vi "ROI entry-Previous ROI compat-Motor Z check.vi"(8 "error in (no error)":errorcluster, 9 "Proceed":bool=TRUE, 10 "ROI fit info cluster in":T1 {"ROI fit info"."Frame size"."Old" items=["100X100"=100, "128X128"=128, "200X200"=200, "256X256"=256, "512X512"=512, "1024x1024"=1024, "2048x2048"=2048]; "ROI fit info"."Frame size"."New" items=["100X100"=100, "128X128"=128, "200X200"=200, "256X256"=256, "512X512"=512, "1024x1024"=1024, "2048x2048"=2048]}, 11 "Old ROI file path":path) -> (0 "error out":errorcluster, 1 "Proceed":bool, 2 "ROI fit info cluster":T1 {"ROI fit info"."Frame size"."Old" items=["100X100"=100, "128X128"=128, "200X200"=200, "256X256"=256, "512X512"=512, "1024x1024"=1024, "2048x2048"=2048]; "ROI fit info"."Frame size"."New" items=["100X100"=100, "128X128"=128, "200X200"=200, "256X256"=256, "512X512"=512, "1024x1024"=1024, "2048x2048"=2048]}, 3 "Old ROI file path (dup)":path)   [LabVIEW 2017]
uses:
  Typedefs/ROI fitting info cluster.ctl
  Typedefs/Frame Size.ctl
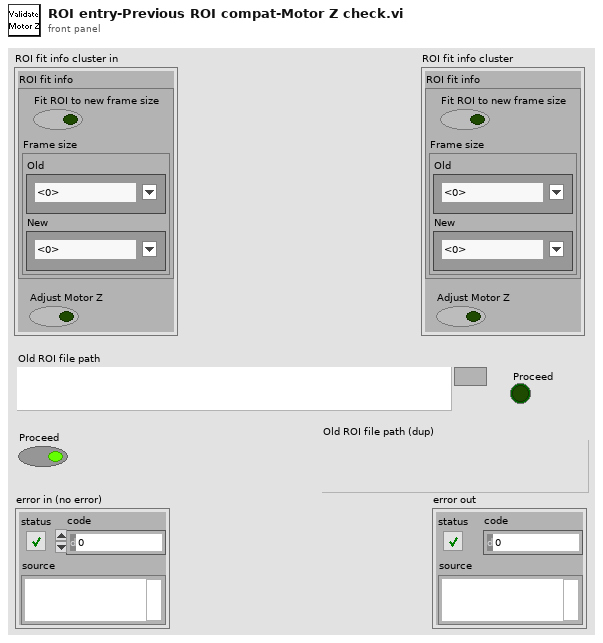
[diagram p1: front panel]
types:
  T1 = typedef "ROI fitting info cluster.ctl" = cluster{"ROI fit info":cluster{"Fit ROI to new frame size":bool, "Frame size":cluster{"Old":T2, "New":T2}}, "Adjust Motor Z":bool}
  T2 = typedef "Frame Size.ctl" = u16
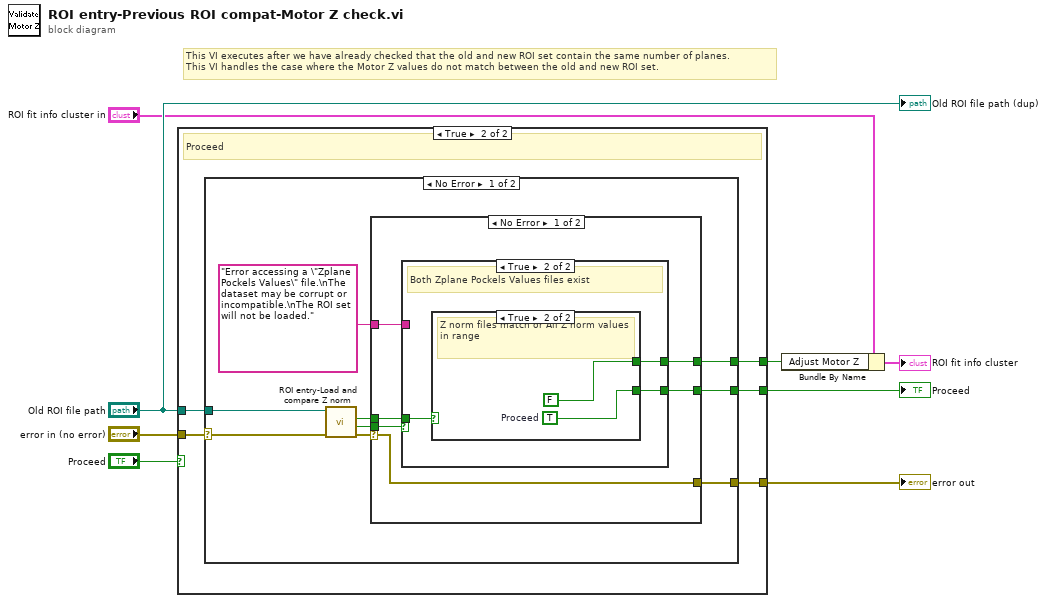
[diagram p0: block diagram]
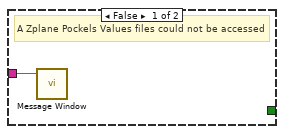
[diagram p3: hidden frame]
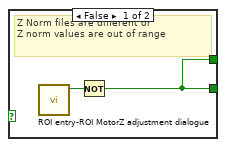
[diagram p4: hidden frame]
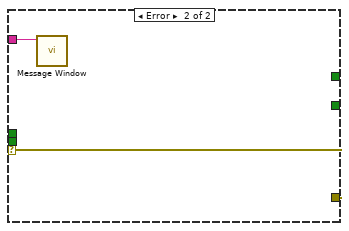
[diagram p5: hidden frame]
diagram:
  # "This VI executes after we have already checked that the old and new ROI set contain the same number of planes.\nThis VI handles the case where the Motor Z values do not match between the old and new ROI set."
  n1 = case shown="True" "Proceed" {
    tunnel: "Old ROI file path" -> [_ w14]
    tunnel: [w9 w13] -> w8
    tunnel: "error in (no error)" -> [w9 w12]
    tunnel: [_ w11] -> w6
    tunnel: [_ w10] -> w1
    frame False {
      # "Skip"
    }
    frame True {
      # "Proceed"
      n2 = case shown="No Error" w12 {
        selector: w12 -> [w20 w40]
        tunnel: w14 -> [w15 _]
        tunnel: [w23 _] -> w11
        tunnel: [w22 w40] -> w13
        tunnel: [w16 _] -> w10
        frame No Error {
          n3 = call "ROI entry-Load and compare Z norm.vi"("error in (no error)"=w20, "Old ROI file path"=w15) -> ("error out"=w19:errorcluster, "Both Zplane Pockels Values files exist"=w18:bool, "All Z values in range"=w17:bool)  [unwired: 3 in, 4 out]
          n4 = case shown="No Error" w19 {
            selector: w19 -> [w24 w39]
            tunnel: w18 -> [w29 _]
            tunnel: [w28 _] -> w23
            tunnel: [w24 w39] -> w22
            tunnel: "Error accessing a \"Zplane Pockels Values\" file.\nThe dataset may be corrupt or incompatible.\nThe ROI set will not be loaded." ("Message string") -> [w27 w38]
            tunnel: w17 -> [w26 _]
            tunnel: [w25 _] -> w16
            frame No Error {
              n5 = case shown="True" w29 {
                tunnel: [_ w31] -> w28
                tunnel: w27 -> [w30 _]
                tunnel: w26 -> [_ w33]
                tunnel: [_ w32] -> w25
                frame False {
                  # "A Zplane Pockels Values files could not be accessed"
                  n6 = call "Message Window.vi"("Message string"=w30) -> ()  [unwired: 10 in, 1 out]
                }
                frame True {
                  # "Both Zplane Pockels Values files exist"
                  n7 = case shown="True" w33 {
                    tunnel: [w34 FALSE] -> w32
                    tunnel: [w34 w37] -> w31
                    frame False {
                      # "Z Norm files are different or\nZ norm values are out of range"
                      n8 = call "ROI entry-ROI MotorZ adjustment dialogue.vi"() -> ("Cancelled (Left button pressed)"=w35:bool)  [unwired: 11 in]
                      n9 = Not(x=w35) -> (.not. x?=w34:bool)
                    }
                    frame True {
                      w37 = TRUE  # Proceed
                      # "Z norm files match or All Z norm values in range"
                    }
                  }
                }
              }
            }
            frame Error {
              n10 = call "Message Window.vi"("Message string"=w38) -> ()  [unwired: 10 in, 1 out]
            }
          }
        }
        frame Error {
        }
      }
    }
  }
  "error out" <- w8
  "Proceed" <- w6
  n11 = Bundle By Name(cluster="ROI fit info cluster in", "Adjust Motor Z"=w1) -> (→"ROI fit info cluster":T1)
  "Old ROI file path (dup)" <- "Old ROI file path"
